vi "CalculateSMax.vi"(8 "error in (no error)":errorcluster, 9 "pair waveform":waveform(sgl), 10 "pair waveform found":bool, 11 "Waveform":waveform(sgl)) -> (0 "error out":errorcluster, 3 "Smax":dbl)   [LabVIEW 2017, in "AnalysisHelper.lvlib"]
uses:
  <vilib>/addons/InsightCM/Utilities/Analysis/Shared/AnalysisHelper.lvlib
  <vilib>/addons/InsightCM/Utilities/Analysis/Vibration/VibrationAnalysisFunctions.lvlib
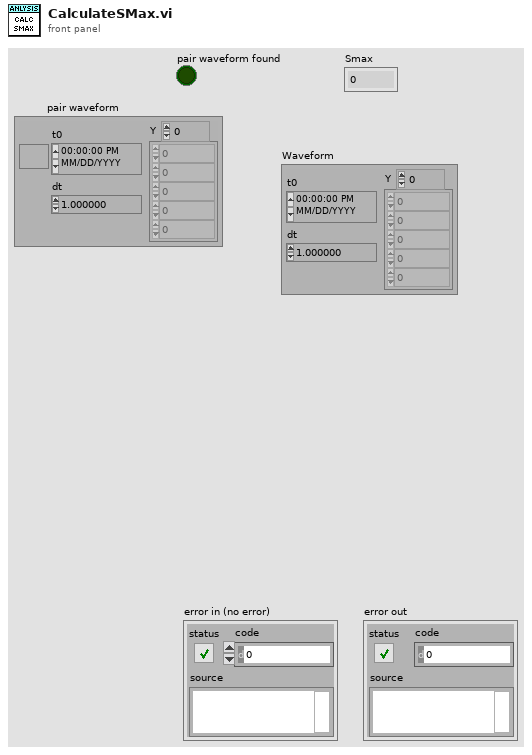
[diagram p1: front panel]
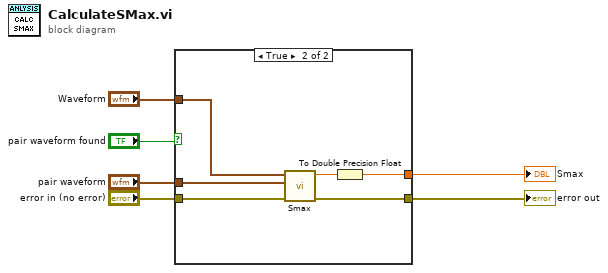
[diagram p0: block diagram]
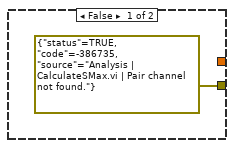
[diagram p2: hidden frame]
diagram:
  n1 = case shown="True" "pair waveform found" {
    tunnel: [errorcluster {"status"=TRUE, "code"=-386735, "source"="Analysis | CalculateSMax.vi | Pair channel not found."} ("error out") w10] -> w3
    tunnel: "error in (no error)" -> [_ w13]
    tunnel: "pair waveform" -> [_ w11]
    tunnel: "Waveform" -> [_ w12]
    tunnel: [_ w8] -> w5
    frame False {
    }
    frame True {
      n2 = call <vilib>:"Smax.vi"("error in ( error)"=w13, "Pair Channel"=w11, "Data"=w12) -> ("error out"=w10:errorcluster, "Smax"=w9:sgl)  [unwired: 7 in]
      n3 = To Double Precision Float(number=w9) -> (double precision float=w8:dbl)
    }
  }
  "Smax" <- w5
  "error out" <- w3
